vi "WT500 Initialize.vi"(0 "VISA resource name":refnum<visa-resource-name>="WT500", 1 "V Range (8: 1000V)":u16(ring)=6 items=["AUTO", "15", "30", "60", "100", "150", "300", "600", "1000", "7.5", "15", "30", "50", "75", "150", "300", "500"], 2 "I Range (7: 40A)":u16(ring)=7 items=["AUTO", "500 mA", "1 A", "2 A", "5 A", "10 A", "20 A", "40 A", "S-AUTO", "50 mV", "100 mV", "200 mV", "500 mV", "1 V", "2 V", "5 V", "10 V", "250 mA", "500 mA", "1 A", "2.5 A", "5 A", "10 A", "20 A", "25 mV", "50 mV", "100 mV", "250 mV", "500 mV", "1 V", "2.5 V", "5 V"], 3 "Error In (No Error) 2":errorcluster) -> (6 "Label":string[](array[string]), 7 "VISA resource name out":refnum<visa-resource-name>="WT500", 10 "Error Out":errorcluster)   [LabVIEW 2016]
uses:
  Type Definitions/WT500 Pole.ctl
  Type Definitions/WT500 Measurements.ctl
  LLBs/ykwt500.llb/YKWT500 Configure Numeric Item (Set).vi
panel:
  in  "Measurement":u16(ring)=1 items=["None", "Urms", "Umn", "Udc", "Urmn", "Uac", "Irms", "Imn", "Idc", "Irmn", "Iac", "P", "S", "Q", "Lambda", "Phi", "Freq U", "Freq I", "U +peak", "U -peak", "I +peak", "I -peak", "Cf U", "Cf I", "Time", "Wp", "Wp+", "Wp-", "q", "q+", "q-", "WS", "WQ", "Eta 1", "Eta 2", "F1", "F2", "F3", "F4", "F5", "F6", "F7", "F8", "U(k)", "I(k)", "P(k)", "S(k)", "Q(k)", "Lambda(k)", "Phi(k)", "Phi U(k)", "Phi I(k)", "Uhdf(k)", "Ihdf(k)", "Phdf(k)", "Uthd", "Ithd", "Pthd", "Phi Ui-Uj", "Phi Ui-Uk", "Phi Ui-Ii", "Phi Ui-Ij", "Phi Ui-Ik", "Delta 1", "Delta 2", "Delta 3", "Delta 4"]
  in  "Pole":u16(ring)=1 items=["NONE", "Element 1", "Element 2", "Element 3", "Sigma"]
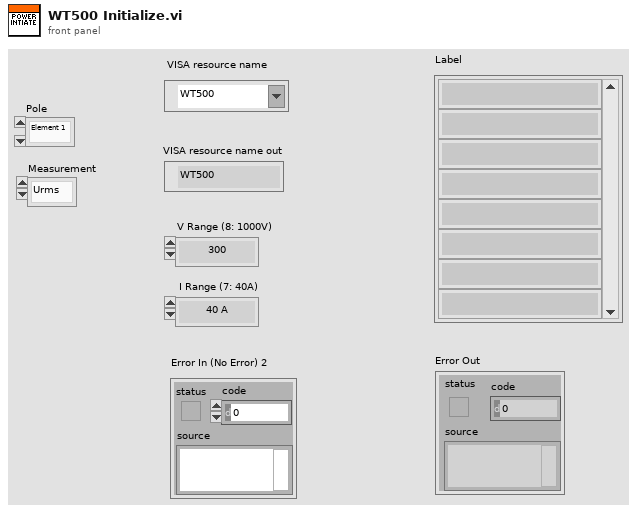
[diagram p1: front panel]
types:
  T1 = typedef "WT500 Measurements.ctl" = u16[]
  T2 = typedef "WT500 Pole.ctl" = u16[]
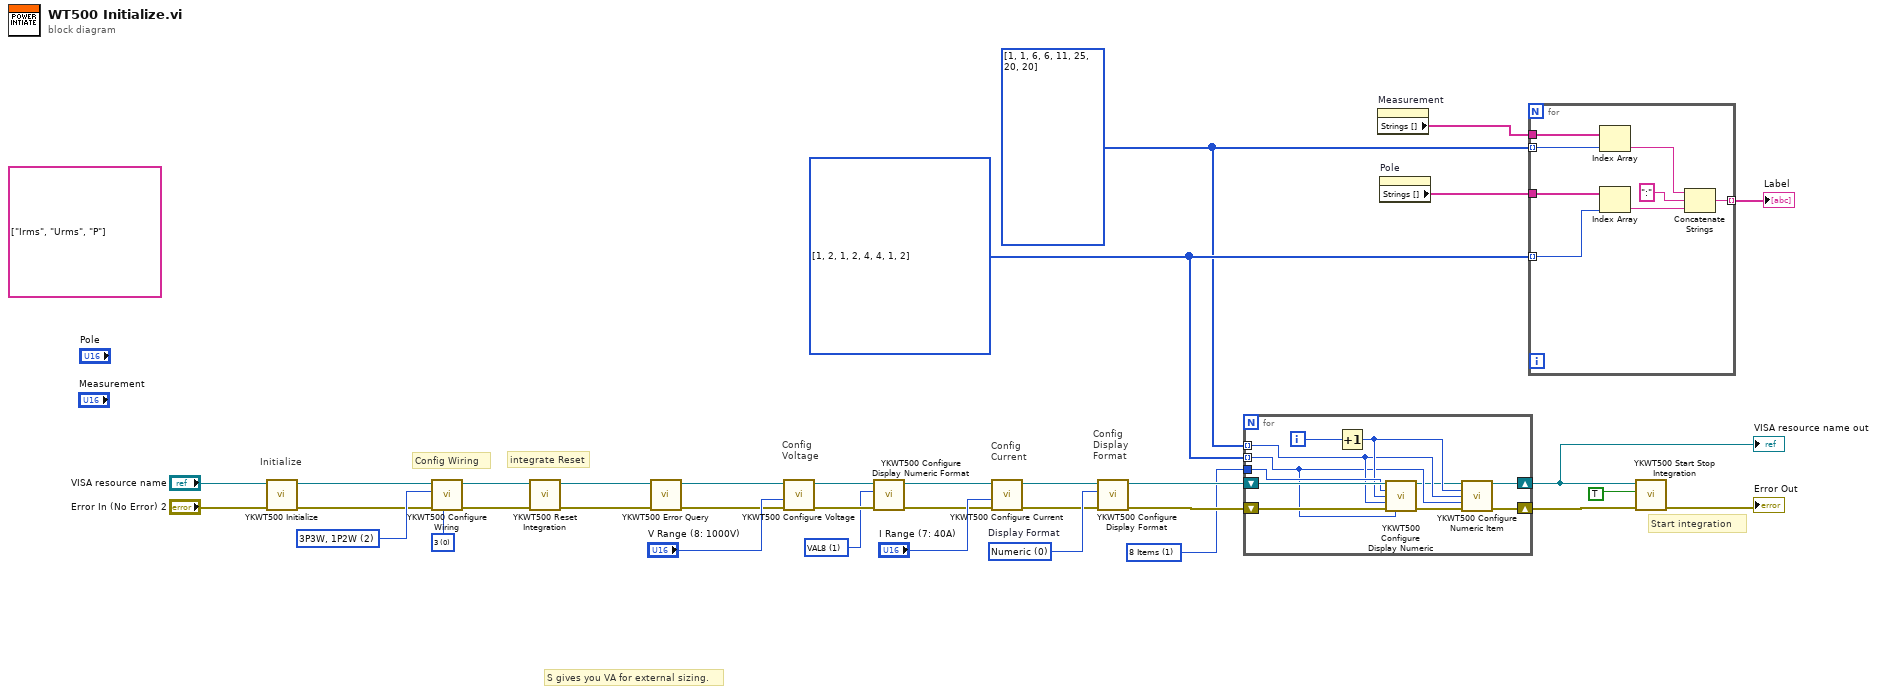
[diagram p0: block diagram]
diagram:
  (unwired) string[] ["Irms", "Urms", "P"]
  w1 = T1 [1, 1, 6, 6, 11, 25, 20, 20] items=["None", "Urms", "Umn", "Udc", "Urmn", "Uac", "Irms", "Imn", "Idc", "Irmn", "Iac", "P", "S", "Q", "Lambda", "Phi", "Freq U", "Freq I", "U +peak", "U -peak", "I +peak", "I -peak", "Cf U", "Cf I", "Time", "Wp", "Wp+", "Wp-", "q", "q+", "q-", "WS", "WQ", "Eta 1", "Eta 2", "F1", "F2", "F3", "F4", "F5", "F6", "F7", "F8", "U(k)", "I(k)", "P(k)", "S(k)", "Q(k)", "Lambda(k)", "Phi(k)", "Phi U(k)", "Phi I(k)", "Uhdf(k)", "Ihdf(k)", "Phdf(k)", "Uthd", "Ithd", "Pthd", "Phi Ui-Uj", "Phi Ui-Uk", "Phi Ui-Ii", "Phi Ui-Ij", "Phi Ui-Ik", "Delta 1", "Delta 2", "Delta 3", "Delta 4"] ("Array of Measurements")
  w17 = u16 0 items=["3", "6"] ("Crest Factor (0: 3)")
  w18 = u16 2 items=["1P2W, 1P2W, 1P2W", "1P3W, 1P2W", "3P3W, 1P2W", "1P2W, 1P3W", "1P2W, 3P3W", "3P4W", "3V3A"] ("Wiring (0: 1P2W, 1P2W, 1P2W)")
  w19 = T2 [1, 2, 1, 2, 4, 4, 1, 2] items=["NONE", "Element 1", "Element 2", "Element 3", "Sigma"]
  w22 = u16 1 items=["VAL4", "VAL8", "VAL16", "MATRIX", "ALL"] ("Display Format (0: Numeric)")
  w27 = u16 1 items=["4 Items", "8 Items", "16 Items", "Matrix"] ("Numeric Format (0: 4 Items)")
  w34 = u16 0 items=["Numeric", "Wave", "Bar", "Vector", "Trend"]  # Display Format
  # "Start integration"
  # "integrate Reset"
  # "Config Wiring"
  # "S gives you VA for external sizing."
  # "Config\nDisplay\nFormat"
  # "Config\nCurrent"
  # "Config\nVoltage"
  # "Initialize"
  n1 = call "YKWT500 Initialize.vi"("error in (no error)"="Error In (No Error) 2", "VISA resource name"="VISA resource name") -> ("error out"=w16:errorcluster, "VISA resource name out"=w9:refnum<visa-resource-name>)  [unwired: 7 in, 1 out]
  n2 = call "YKWT500 Configure Wiring.vi"("Crest Factor (0: 3)"=w17, "error in (no error)"=w16, "Wiring (0: 1P2W, 1P2W, 1P2W) 2"=w18, "VISA resource name"=w9) -> ("error out"=w15:errorcluster, "VISA resource name out"=w14:refnum<visa-resource-name>)  [unwired: 6 in]
  n3 = call "YKWT500 Reset Integration.vi"("error in (no error)"=w15, "VISA resource name"=w14) -> ("error out"=w12:errorcluster, "VISA resource name out"=w13:refnum<visa-resource-name>)  [unwired: 8 in]
  n4 = call "YKWT500 Error Query.vi"("error in (no error)"=w12, "VISA resource name"=w13) -> ("error out"=w20:errorcluster, "VISA resource name out"=w21:refnum<visa-resource-name>)  [unwired: 6 in, 2 out]
  n5 = call "YKWT500 Configure Voltage.vi"("error in (no error)"=w20, "Voltage Range (8: 1000V)"="V Range (8: 1000V)", "VISA resource name"=w21) -> ("error out"=w26:errorcluster, "VISA resource name out"=w23:refnum<visa-resource-name>)  [unwired: 7 in]
  n6 = call "YKWT500 Configure Display Numeric Format.vi"("error in (no error)"=w26, "Numeric Format (0: 4 Items)"=w22, "VISA resource name"=w23) -> ("error out"=w25:errorcluster, "VISA resource name out"=w24:refnum<visa-resource-name>)  [unwired: 7 in]
  n7 = call "YKWT500 Configure Current.vi"("error in (no error)"=w25, "Current Range (7: 40A)"="I Range (7: 40A)", "VISA resource name"=w24) -> ("error out"=w33:errorcluster, "VISA resource name out"=w32:refnum<visa-resource-name>)  [unwired: 7 in]
  n8 = call "YKWT500 Configure Display Format.vi"("error in (no error)"=w33, "Display Format (0: Numeric)"=w34, "VISA resource name"=w32) -> ("error out"=w28:errorcluster, "VISA resource name out"=w29:refnum<visa-resource-name>)  [unwired: 7 in]
  n9 = for {
    shift-right: [w37] -> w5
    shift-left: w29 -> [w45]
    shift-right: [w35] -> w10
    shift-left: w28 -> [w44]
    tunnel: w27 -> [w42]
    tunnel: w19 -> [w39] mode=indexing
    tunnel: w1 -> [w40] mode=indexing
    i -> [w43]
    n10 = Increment(x=w43) -> (x+1=w41:i32)
    n11 = call "YKWT500 Configure Display Numeric.vi"("VISA resource name"=w45, "Numeric Format (0: 4 Items)"=w42, "Numeric Item Number (1)"=w41, "Numeric Function (0: None)"=w40, "error in (no error)"=w44, "Element (1: Element 1)"=w39) -> ("VISA resource name out"=w38:refnum<visa-resource-name>, "error out"=w36:errorcluster)  [unwired: 8 in]
    n12 = call-poly "YKWT500 Configure Numeric Item.vi"("VISA resource name"=w38, "Numeric Item Number (1)"=w41, "Numeric Function (0: None)"=w40, "Element (1: Element 1)"=w39, "error in (no error)"=w36) -> ("VISA resource name out"=w37:refnum<visa-resource-name>, "error out"=w35:errorcluster)  [unwired: 9 in]
  }
  "VISA resource name out" <- w5
  n13 = property on="Measurement" class="Ring (strict)"() -> ("Strings []"=w4:string[])  [unwired: 2 in, 2 out]
  n14 = property on="Pole" class="Ring (strict)"() -> ("Strings []"=w3:string[])  [unwired: 2 in, 2 out]
  n15 = for {
    tunnel: w1 -> [w46] mode=indexing
    tunnel: w4 -> [w53]
    tunnel: w19 -> [w47] mode=indexing
    tunnel: w3 -> [w52]
    tunnel: [w48] -> w2 mode=indexing
    n16 = Index Array(array=w53, index=w46) -> (element=w51:string)
    n17 = Index Array(array=w52, index=w47) -> (element=w49:string)
    n18 = Concatenate Strings(w51, ":" ("string"), w49) -> (w48:string)
  }
  "Label" <- w2
  n19 = call "YKWT500 Start Stop Integration.vi"("error in (no error)"=w10, "Start/Stop (False: Stop)"=TRUE, "VISA resource name"=w5) -> ("error out"=→"Error Out":errorcluster)  [unwired: 7 in, 1 out]
